vi "Add Plugin.vi"(10 "Menu in":refnum<class "MGI_Menu.lvclass">, 11 "Active Plugins in":refnum<class "MGI_Plugin.lvclass">[](array[class])) -> (2 "Menu out":refnum<class "MGI_Menu.lvclass">, 3 "Active Plugins out":refnum<class "MGI_Plugin.lvclass">[](array[class]))   [LabVIEW 2016]
uses:
  <userlib>/_MGI/Menu Building/Example/Plugin/MGI_Plugin.lvclass
  <userlib>/_MGI/Menu Building/MenuTypes/MGI_Menu.lvclass
  <userlib>/_MGI/Menu Building/MenuTypes/Read Menu Items.vi
  <userlib>/_MGI/Menu Building/MenuItem/MenuItem.vi
  <userlib>/_MGI/Menu Building/MenuItem/Read Sub-Menus.vi
  <userlib>/_MGI/Menu Building/MenuItem/Write Sub-Menus.vi
  <userlib>/_MGI/Menu Building/MenuItem/MGI_MenuItem.lvclass
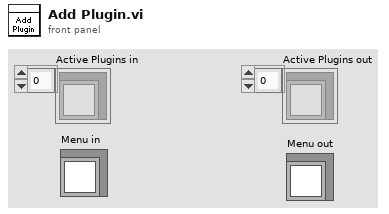
[diagram p1: front panel]
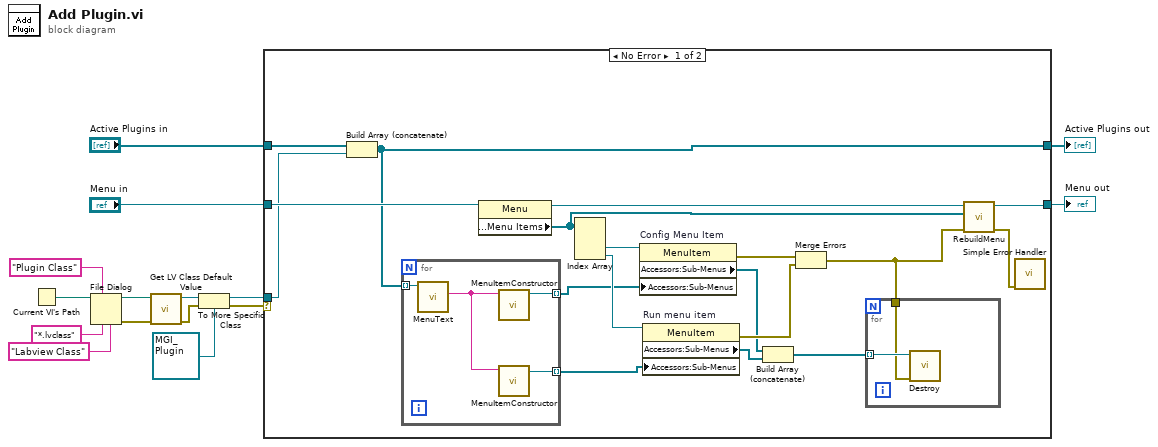
[diagram p0: block diagram]
diagram:
  n1 = Current VI's Path() -> (path=w1:path)
  n2 = File Dialog(4:"Labview Class" ("pattern label"), 6:"*.lvclass" ("pattern (all files)"), 7:"Plugin Class" ("prompt"), 11:w1) -> (0:w2:errorcluster, 3:w6:path)  [unwired: 3 in, 2 out]
  n3 = call <vilib>:"Get LV Class Default Value.vi"("error in (no error)"=w2, "class path"=w6) -> ("error out"=w13:errorcluster, "object"=w15:refnum<class>)  [unwired: 8 in]
  n4 = To More Specific Class(target class=refnum<class "MGI_Plugin.lvclass"> refnum ("Plugin.lvclass"), reference=w15, error in=w13) -> (specific class reference=w11:refnum<class "MGI_Plugin.lvclass">, error out=w12:errorcluster)
  n5 = case shown="No Error" w12 {
    tunnel: "Active Plugins in" -> [w33 w41]
    tunnel: [w29 w41] -> w7
    tunnel: w11 -> [w30 _]
    tunnel: "Menu in" -> [w32 w40]
    tunnel: [w31 w40] -> w9
    frame No Error {
      n6 = Build Array (concatenate)(w33, w30) -> (w29:refnum<class "MGI_Plugin.lvclass">[])
      n7 = for {
        tunnel: w29 -> [w39] mode=indexing
        tunnel: [w38] -> w22 mode=indexing
        tunnel: [w37] -> w21 mode=indexing
        n8 = call-dynamic "MenuText.vi"("MGI_Plugin.lvclass"=w39) -> ("Menu Text"=w36:string)  [unwired: 8 in, 2 out]
        n9 = call-poly <userlib>:"MenuItemConstructor.vi"("Text"=w36) -> ("MenuItem"=w38:refnum<data-value>)  [unwired: 9 in, 1 out]
        n10 = call-poly <userlib>:"MenuItemConstructor.vi"("Text"=w36) -> ("MenuItem"=w37:refnum<data-value>)  [unwired: 9 in, 1 out]
      }
      n11 = property class="Menu"(reference=w32) -> (reference out=w26:refnum<class "MGI_Menu.lvclass">, "Accessors:Menu Items"=w25:refnum<data-value>[])  [unwired: 1 in, 1 out]
      n12 = Index Array(array=w25) -> (element #2=w28:refnum<data-value>, element #3=w27:refnum<data-value>)  [unwired: 3 in, 1 out]
      n13 = property on="Config Menu Item" class="MenuItem"(reference=w28, "Accessors:Sub-Menus"=w22) -> (error out=w24:errorcluster, "Accessors:Sub-Menus"=w20:refnum<data-value>[])  [unwired: 1 in, 1 out]
      n14 = property on="Run menu item" class="MenuItem"(reference=w27, "Accessors:Sub-Menus"=w21) -> (error out=w23:errorcluster, "Accessors:Sub-Menus"=w19:refnum<data-value>[])  [unwired: 1 in, 1 out]
      n15 = Build Array (concatenate)(w20, w19) -> (w18:refnum<data-value>[])
      n16 = Merge Errors(w24, w23) -> (w16:errorcluster)
      n17 = for {
        tunnel: w18 -> [w35] mode=indexing
        tunnel: w16 -> [w34]
        n18 = call <userlib>:"Destroy.vi"("error in (no error)"=w34, "Menu Item ref"=w35) -> ()  [unwired: 9 in, 1 out]
      }
      n19 = call <userlib>:"RebuildMenu.vi"("error in (no error)"=w16, "New Menu Items"=w25, "Menu in"=w26) -> ("error out"=w17:errorcluster, "Menu out"=w31:refnum<class "MGI_Menu.lvclass">)  [unwired: 7 in]
      n20 = call <vilib>:"Simple Error Handler.vi"("error in (no error)"=w17) -> ()  [unwired: 4 in, 5 out]
    }
    frame Error {
    }
  }
  "Active Plugins out" <- w7
  "Menu out" <- w9
